vi "MeasureMagnetoCaloric_wendel.vi"   [LabVIEW 2019]
uses:
  Global/Global Variables/global.vi
  Monitors/Utility/Monitor Communication/AMI/AMI_Control.ctl
  Global/Global Variables/Data_Display_global.vi
types:
  T1 = typedef "AMI_Control.ctl" = cluster{"B AMI rate (T)":dbl, "AMI Set field":bool, "B AMI Setpoint (T)":dbl, "Phi AMI Setpoint (Deg) ":dbl, "Switch Heater":bool, "Y-Axis Setpoint (T)":dbl, "Y-Axis Rate (T/min)":dbl, "Z-Axis Setpoint (T)":dbl, "Z-Axis Rate (T/min)":dbl}
  T2 = typedef "AMI_cluster.ctl" = cluster{"Y Axis Status":enum16{"", "RAMPING", "HOLDING", "PAUSED", "MANUAL UP", "MANUAL DOWN", "ZEROING CURRENT", "QUENCH DETECTED", "HEATING SWITCH", "AT ZER0", "COOLING SWITCH"}, "Z Axis Status":enum16{"", "RAMPING", "HOLDING", "PAUSED", "MANUAL UP", "MANUAL DOWN", "ZEROING CURRENT", "QUENCH DETECTED", "HEATING SWITCH", "AT ZER0", "COOLING SWITCH"}, "Y-Axis (T)":dbl, "Y-Axis Setpoint (T)":dbl, "Y-Axis Rate (T/min)":dbl, "Z-Axis (T)":dbl, "Z-Axis Setpoint (T)":dbl, "Z-Axis Rate (T/min)":dbl, "B AMI rate (T)":dbl, "AMI Monitor":bool, "AMI Set field rates":bool, "AMI Set field":bool, "Switch Heater Y":bool, "Switch Heater Z":bool, "Switch Heater":bool, "B AMI (T)":dbl, "B AMI Setpoint (T)":dbl, "Phi AMI (Deg) ":dbl, "Phi AMI Setpoint (Deg) ":dbl}
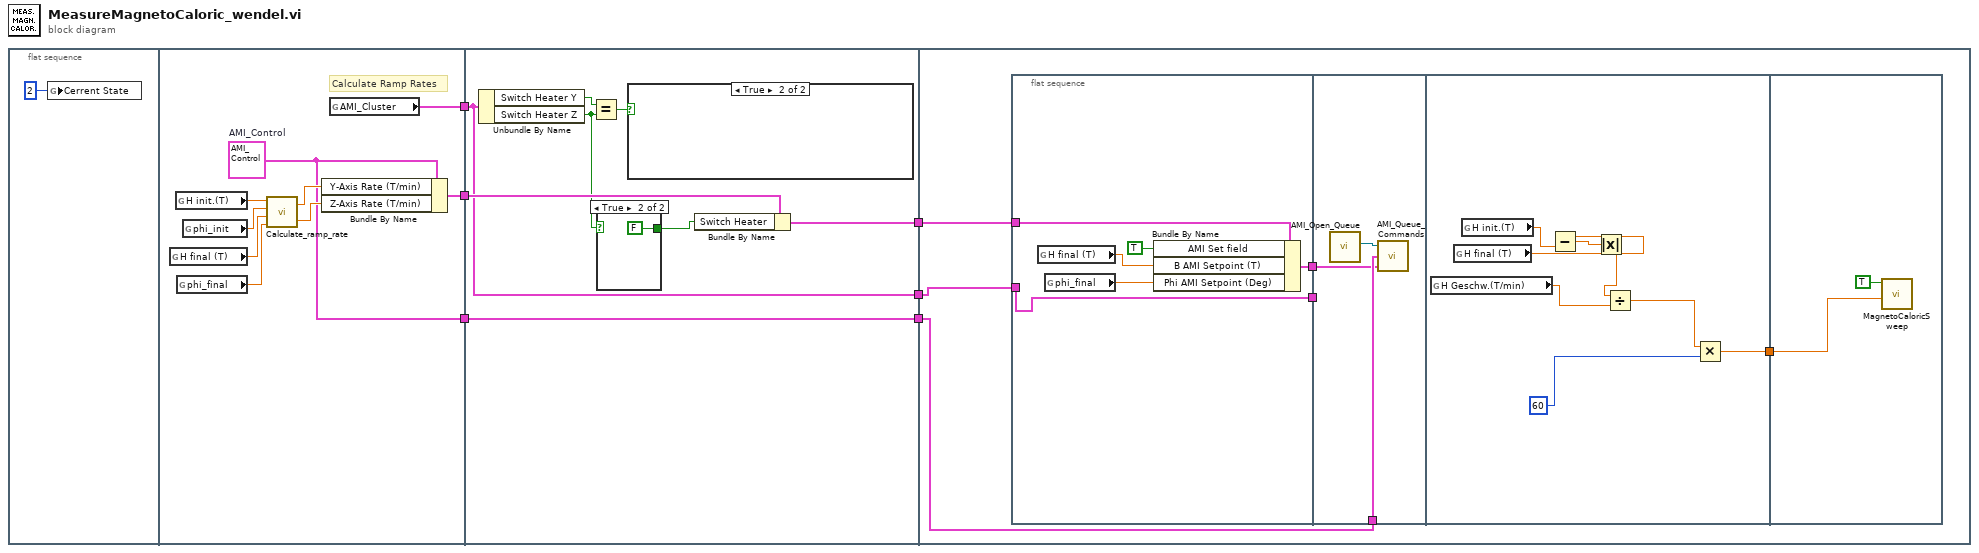
[diagram p0: block diagram]
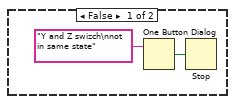
[diagram p2: hidden frame]
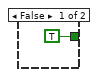
[diagram p3: hidden frame]
diagram:
  n1 = flat-sequence {
    tunnel: [w14] -> w6
    tunnel: [w9] -> w2
    tunnel: [w8] -> w1
    tunnel: w6 -> [w17]
    tunnel: [w17] -> w5
    tunnel: [w23] -> w4
    tunnel: [w21] -> w3
    tunnel: w2 -> [w22]
    tunnel: w1 -> [w21]
    tunnel: w5 -> [w31]
    tunnel: w4 -> [w34]
    tunnel: w3 -> [w30]
    frame #0 {
      n2 = global write "global.vi" "Cerrent State"(2) -> ()
    }
    frame #1 {
      w8 = T1 {"B AMI rate (T)"=0.0, "AMI Set field"=FALSE, "B AMI Setpoint (T)"=0.0, "Phi AMI Setpoint (Deg) "=0.0, "Switch Heater"=FALSE, "Y-Axis Setpoint (T)"=0.0, "Y-Axis Rate (T/min)"=0.0, "Z-Axis Setpoint (T)"=0.0, "Z-Axis Rate (T/min)"=0.0}  # AMI_Control
      # "Calculate Ramp Rates"
      n3 = global read "global.vi" "H final (T)"() -> (w16:dbl)
      n4 = global read "global.vi" "H init.(T)"() -> (w11:dbl)
      n5 = global read "global.vi" "phi_final"() -> (w15:dbl)
      n6 = global read "global.vi" "phi_init"() -> (w10:dbl)
      n7 = call "Calculate_ramp_rate.vi"("Phi (Deg)"=w15, "H_final (T)"=w16, "Phi_init (Deg)"=w10, "H_init (T)"=w11) -> ("Z-Ramp"=w13:dbl, "Y-Ramp"=w12:dbl)  [unwired: 2 in]
      n8 = Bundle By Name(cluster=w8, "Y-Axis Rate (T/min)"=w12, "Z-Axis Rate (T/min)"=w13) -> (w9:T1)
      n9 = global read "Data_Display_global.vi" "AMI_Cluster"() -> (w14:T2)
    }
    frame #2 {
      n10 = Unbundle By Name(w17) -> ("Switch Heater Y"=w20:bool, "Switch Heater Z"=w19:bool)
      n11 = Equal?(x=w20, y=w19) -> (x = y?=w18:bool)
      n12 = case shown="True" w19 {
        tunnel: [TRUE FALSE] -> w24
        frame False {
        }
        frame True {
        }
      }
      n13 = case shown="True" w18 {
        frame False {
          n14 = One Button Dialog(message="Y and Z swizch\nnot in same state") -> (true=w25:bool)  [unwired: 1 in]
          n15 = Stop(stop? (T)=w25) -> ()
        }
        frame True {
        }
      }
      n16 = Bundle By Name(cluster=w22, "Switch Heater"=w24) -> (w23:T1)
    }
    frame #3 {
      n17 = flat-sequence {
        tunnel: w34 -> [w40]
        tunnel: [w36] -> w33
        tunnel: [w35] -> w32
        tunnel: w31 -> [w35]
        tunnel: w33 -> [w41]
        tunnel: w32 -> [_]
        tunnel: w30 -> [w42]
        tunnel: [w44] -> w29
        tunnel: w29 -> [w52]
        frame #0 {
          n18 = global read "global.vi" "H final (T)"() -> (w38:dbl)
          n19 = global read "global.vi" "phi_final"() -> (w39:dbl)
          n20 = Bundle By Name(cluster=w40, "AMI Set field"=TRUE, "B AMI Setpoint (T)"=w38, "Phi AMI Setpoint (Deg)"=w39) -> (w36:T1)
        }
        frame #1 {
          n21 = call "AMI_Open_Queue.vi"() -> ("queue out"=w43:refnum<queue>)  [unwired: 10 in, 1 out]
          n22 = call "AMI_Queue_Commands.vi"("AMI_Control"=w41, "Last Status"=w42, "Queue in"=w43) -> ()  [unwired: 1 out]
        }
        frame #2 {
          n23 = global read "global.vi" "H Geschw.(T/min)"() -> (w47:dbl)
          n24 = global read "global.vi" "H final (T)"() -> (w51:dbl)
          n25 = global read "global.vi" "H init.(T)"() -> (w50:dbl)
          n26 = Subtract(x=w51, y=w50) -> (x-y=w49:dbl)
          n27 = Absolute Value(x=w49) -> (abs(x)=w48:dbl)
          n28 = Divide(x=w48, y=w47) -> (x/y=w46:dbl)
          n29 = Multiply(x=w46, y=60) -> (x*y=w44:dbl)
        }
        frame #3 {
          n30 = call "MagnetoCaloricSweep.vi"(9:w52, 11:TRUE) -> ()  [unwired: 10 in]
        }
      }
    }
  }
